vi "Register New DBL Item.vi"(8 "error in (no error)":errorcluster, 9 "element data type":dbl, 10 "Tag Name":string, 11 "Current Value Table in":refnum<class "Current Value Table.lvclass">) -> (0 "error out":errorcluster, 3 "Current Value Table out":refnum<class "Current Value Table.lvclass">)   [LabVIEW 2024, in "Current Value Table.lvlib" / "Current Value Table.lvclass"]
uses:
  Current Value Table.lvclass
  CVT_DBL/CVT_DBL.lvclass
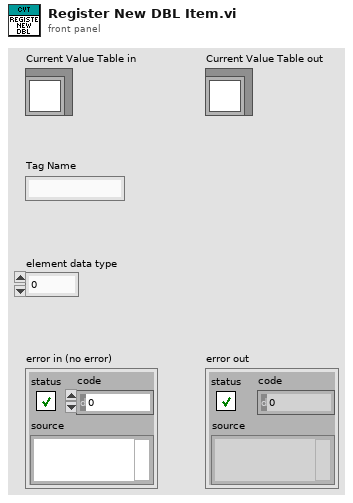
[diagram p1: front panel]
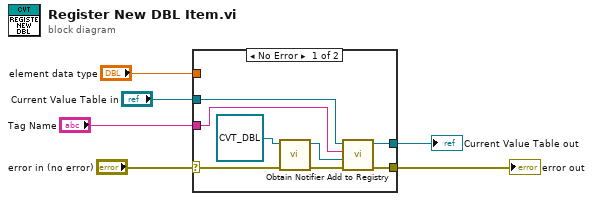
[diagram p0: block diagram]
diagram:
  n1 = case shown="No Error" "error in (no error)" {
    selector: "error in (no error)" -> [w13 w16]
    tunnel: [w7 w16] -> w5
    tunnel: [w11 w15] -> w3
    tunnel: "Current Value Table in" -> [w12 w15]
    tunnel: "Tag Name" -> [w10 _]
    tunnel: "element data type" -> [_ _]
    frame No Error {
      n2 = call-dynamic "Obtain Notifier.vi"("error in (no error)"=w13, "CVT_DBL in"=refnum<class "CVT_DBL.lvclass"> refnum) -> ("error out"=w8:errorcluster, "CVT_DBL out"=w9:refnum<class "CVT_DBL.lvclass">)  [unwired: 8 in]
      n3 = call-dynamic "Add to Registry.vi"("error in (no error)"=w8, "iCVT_Item in"=w9, "Tag Name"=w10, "Current Value Table in"=w12) -> ("error out"=w7:errorcluster, "Current Value Table out"=w11:refnum<class "Current Value Table.lvclass">)  [unwired: 5 in, 1 out]
    }
    frame Error {
    }
  }
  "error out" <- w5
  "Current Value Table out" <- w3
